vi "TabControl.vi"(8 "error in":errorcluster, 11 "Gen Refnum":refnum<vi>) -> (0 "error out":errorcluster, 3 "Tab out":refnum<class "Tab.lvclass">)   [LabVIEW 2014, in "Raspberry Pi Compatible Compiler for LabVIEW.lvlib" / "Tab.lvclass"]
uses:
  Tab.lvclass
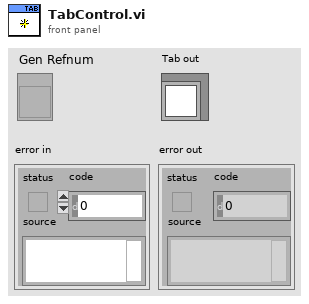
[diagram p1: front panel]
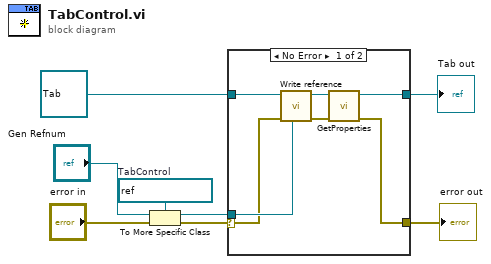
[diagram p0: block diagram]
diagram:
  w8 = refnum<vi> refnum  # TabControl
  n1 = To More Specific Class(target class=w8, reference="Gen Refnum", error in="error in") -> (specific class reference=w6:refnum<vi>, error out=w7:errorcluster)
  n2 = case shown="No Error" w7 {
    selector: w7 -> [w12 w17]
    tunnel: refnum<class "Tab.lvclass"> refnum ("Tab in") -> [w15 w16]
    tunnel: w6 -> [w13 _]
    tunnel: [w10 w16] -> w2
    tunnel: [w9 w17] -> w1
    frame No Error {
      n3 = call-dynamic "Write reference.vi"("reference"=w13, "error in"=w12, "GObject in"=w15) -> ("error out"=w11:errorcluster, "GObject out"=w14:refnum<class "Tab.lvclass">)  [unwired: 5 in]
      n4 = call-dynamic "GetProperties.vi"("error in"=w11, "Tab in"=w14) -> ("error out"=w9:errorcluster, "Tab out"=w10:refnum<class "Tab.lvclass">)  [unwired: 8 in]
    }
    frame Error {
    }
  }
  "error out" <- w1
  "Tab out" <- w2
